vi "FilterSettingsToBandwidth.vi"(9 "Moving Average Enable":bool, 10 "Moving Average Type":u8(ring) items=["40 ns"=1, "80 ns"=2, "160 ns"=3, "320 ns"=4, "640 ns"=5, "1.28 us"=6], 11 "Pre-Filter":u8(ring) items=["None", "20 MHz filter"]) -> (3 "Bandwidth":T1 format="%x")   [LabVIEW 2009]
uses:
  libraries/Cscope control driver.llb/Input Bandwidth.ctl
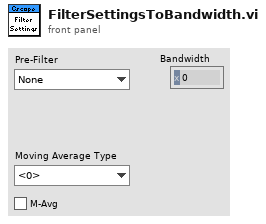
[diagram p1: front panel]
types:
  T1 = typedef "Input Bandwidth.ctl" = u16
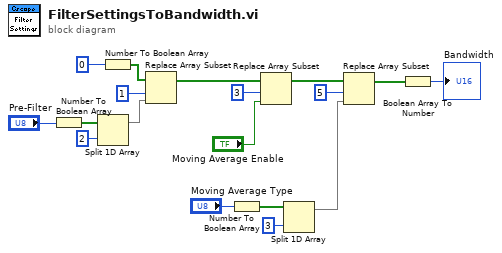
[diagram p0: block diagram]
diagram:
  n1 = Number To Boolean Array(number="Pre-Filter") -> (Boolean array=w11:bool[])
  n2 = Split 1D Array(array=w11, index=2) -> (first subarray=w8:bool[])  [unwired: 1 out]
  n3 = Number To Boolean Array(number=u8 0) -> (Boolean array=w13:bool[])
  n4 = Replace Array Subset(array=w13, new element=w8, index=1) -> (w7:bool[])
  n5 = Number To Boolean Array(number="Moving Average Type") -> (Boolean array=w3:bool[])
  n6 = Replace Array Subset(array=w7, new element="Moving Average Enable", index=3) -> (w6:bool[])
  n7 = Split 1D Array(array=w3, index=3) -> (first subarray=w1:bool[])  [unwired: 1 out]
  n8 = Replace Array Subset(array=w6, new element=w1, index=5) -> (w2:bool[])
  n9 = Boolean Array To Number(Boolean array=w2) -> (number=→"Bandwidth":u32)
